vi "One Button Dialog_TouchScreen.vi"(1 "Button name (\"OK\")":string, 2 "Message":string) -> (0 "true":T1)   [LabVIEW 2010]
uses:
  _TypeDefs/OK Button_TouchScreen.ctl
panel:
  in  "T Button":T1
  out "Message Indicator":string
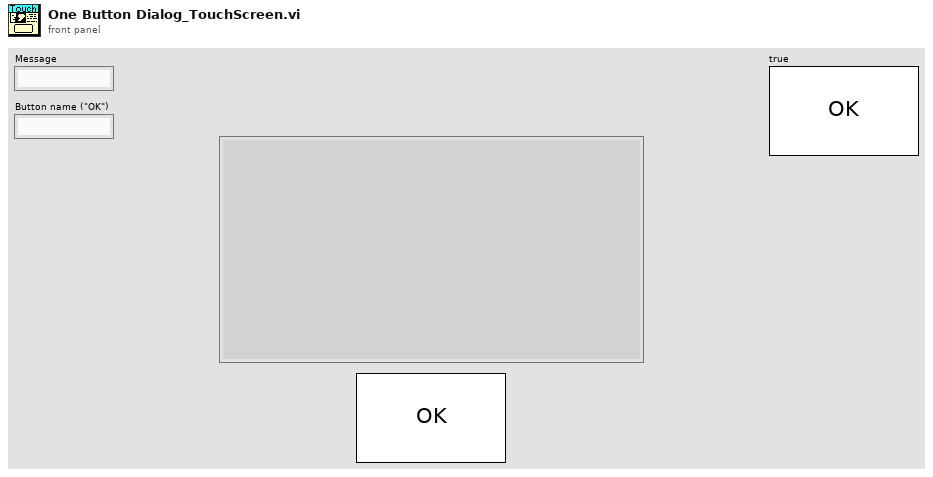
[diagram p1: front panel]
types:
  T1 = typedef "OK Button_TouchScreen.ctl" = bool
  T2 = enum8{"Enabled", "Disabled", "Disabled and Grayed Out"}
  T3 = cluster{"left":i16, "top":i16, "right":i16, "bottom":i16}
  T4 = typedef "LVBoundsTypeDef.ctl" = cluster{"Width":u32, "Height":u32}
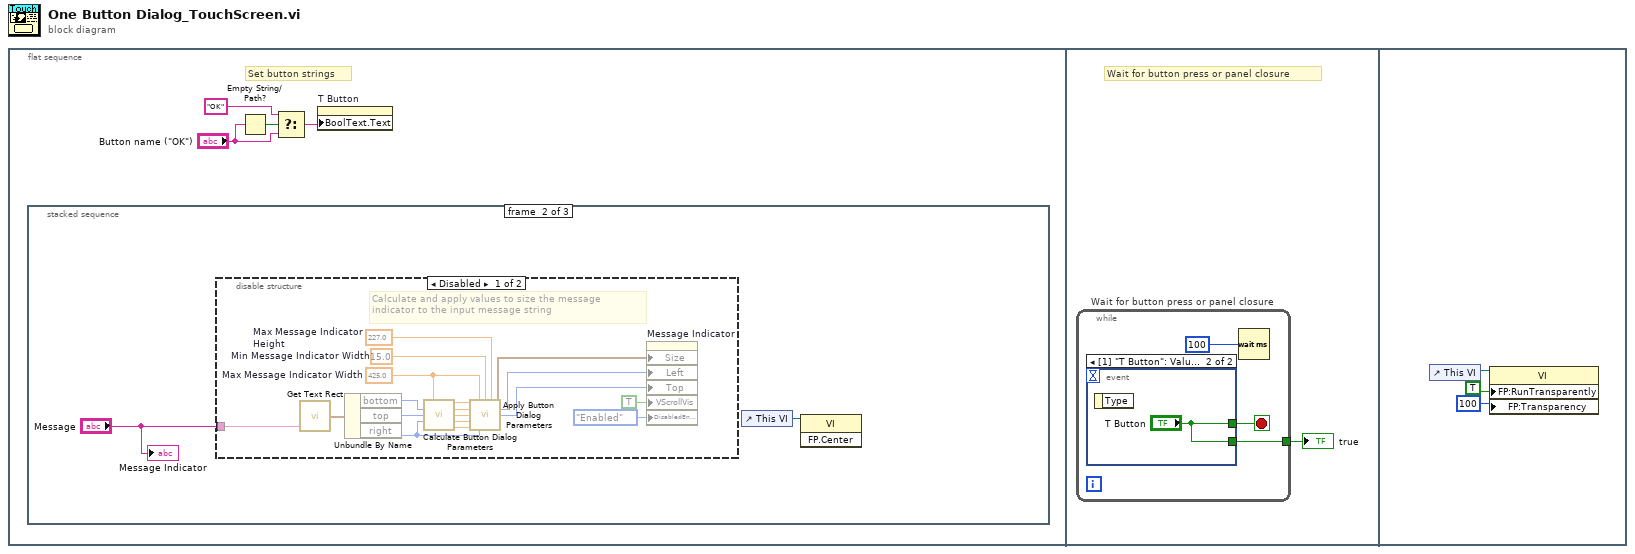
[diagram p0: block diagram]
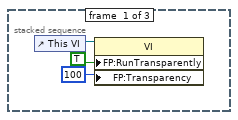
[diagram p2: hidden frame]
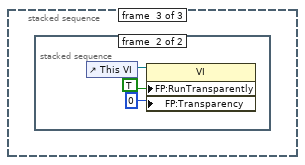
[diagram p4: hidden frame]
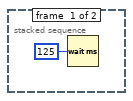
[diagram p5: hidden frame]
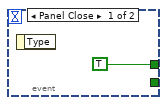
[diagram p6: hidden frame]
diagram:
  n1 = flat-sequence {
    frame #0 {
      # "Set button strings"
      n2 = stacked-sequence {
        frame #0 {
          n3 = control-ref of="This VI"() -> (w5:refnum<vi>)
          n4 = property class="VI"(reference=w5, "FP:RunTransparently"=TRUE, "FP:Transparency"=u8 100 ("Front Panel Window:Transparency")) -> ()  [unwired: 1 in, 2 out]
        }
        frame #1 {
          n5 = disable-structure shown="Disabled" {
            disable-tunnel: "Message" -> [w10 _]
            frame Disabled {
              w19 = 15.0  # Min Message Indicator Width
              w18 = 227.0  # Max Message Indicator Height
              w22 = 425.0  # Max Message Indicator Width
              # "Calculate and apply values to size the message indicator to the input message string"
              n6 = call <vilib>:"Get Text Rect.vi"("text"=w10) -> ("rect"=w26:T3)  [unwired: 8 in]
              n7 = Unbundle By Name(w26) -> ("bottom"=w14:i16, "top"=w15:i16, "right"=w13:i16)
              n8 = call "Calculate Button Dialog Parameters.vi"("Max Message Indicator Width"=w22, "bottom"=w14, "top"=w15, "right"=w13) -> ("Indicator left position"=w23:dbl, "Calculated indicator height"=w21:dbl, "Indicator height scaled large"=w20:dbl, "Actual indicator height"=w17:dbl, "Indicator height scaled small"=w16:dbl)  [unwired: 7 in]
              n9 = call "Apply Button Dialog Parameters.vi"("Indicator left position"=w23, "Max Message Indicator Width"=w22, "Min Message Indicator Width"=w19, "Max Message Indicator Height"=w18, "Calculated indicator height"=w21, "Indicator height scaled large"=w20, "Actual indicator height"=w17, "Indicator height scaled small"=w16, "right"=w13) -> ("Message indicator size"=w27:T4, "Message indicator left"=w25:i32, "Message indicator top"=w24:i32)  [unwired: 1 in, 3 out]
              n10 = property on="Message Indicator" class="Str"("Size"=w27, "Left"=w25, "Top"=w24, "VScrollVis"=TRUE, "DisabledEnum"=T2."Enabled" ("Disabled")) -> ()  [unwired: 2 in, 2 out]
            }
            frame Enabled {
            }
          }
          n11 = control-ref of="This VI"() -> (w8:refnum<vi>)
          n12 = invoke class="VI" method="FP.Center"(reference=w8) -> ()  [unwired: 2 in, 3 out]
          "Message Indicator" <- "Message"
        }
        frame #2 {
          n13 = stacked-sequence {
            frame #0 {
              n14 = Wait (ms)(milliseconds to wait=u32 125) -> ()  [unwired: 1 out]
            }
            frame #1 {
              n15 = control-ref of="This VI"() -> (w31:refnum<vi>)
              n16 = property class="VI"(reference=w31, "FP:RunTransparently"=TRUE, "FP:Transparency"=u8 0 ("Front Panel Window:Transparency")) -> ()  [unwired: 1 in, 2 out]
            }
          }
        }
      }
      n17 = Empty String/Path?(string/path="Button name (\"OK\")") -> (empty?=w4:bool)
      n18 = Select(t="OK", s=w4, f="Button name (\"OK\")") -> (s? t:f=w2:string)
      n19 = property on="T Button" class="Bool"("BoolText.Text"=w2) -> ()  [unwired: 2 in, 2 out]
    }
    frame #1 {
      # "Wait for button press or panel closure"
      n20 = while "Wait for button press or panel closure" {
        tunnel: [w34] -> w32
        stop <- w35 stop-if-true
        n21 = event shown="[1] \"T Button\": Value Change" {
          selector: _ -> [_ _]
          dyn-events: _ -> [_ _]
          timeout: _ -> [_ _]
          tunnel: [T1 TRUE ("T Button") "T Button"] -> w35
          tunnel: [_ "T Button"] -> w34
          event Panel Close {
            n22 = event-data() -> ()  [unwired: 1 in, 1 out]
          }
          event Value Change {
            n23 = event-data() -> ()  [unwired: 1 in, 1 out]
          }
        }
        n24 = Wait (ms)(milliseconds to wait=u32 100) -> ()  [unwired: 1 out]
      }
      "true" <- w32
    }
    frame #2 {
      n25 = control-ref of="This VI"() -> (w40:refnum<vi>)
      n26 = property class="VI"(reference=w40, "FP:RunTransparently"=TRUE, "FP:Transparency"=u8 100 ("Front Panel Window:Transparency")) -> ()  [unwired: 1 in, 2 out]
    }
  }
